vi "sum of N Gaussians with offset model_MODCA.vi"(3 "output control":T1, 4 "data":variant, 5 "X":dbl[](array[numeric]), 6 "a":dbl[](array[numeric])) -> (0 "error out":errorcluster, 1 "f'(X,a)":dbl[][](array[numeric]), 2 "f(X,a)":dbl[](array[numeric]))   [LabVIEW 2020]
doc: "Sum of three Gaussians, plus DC offset."
uses:
  <vilib>/gmath/NumericalOptimization/LM_output select.ctl
  <vilib>/gmath/NI_Gmath.lvlib
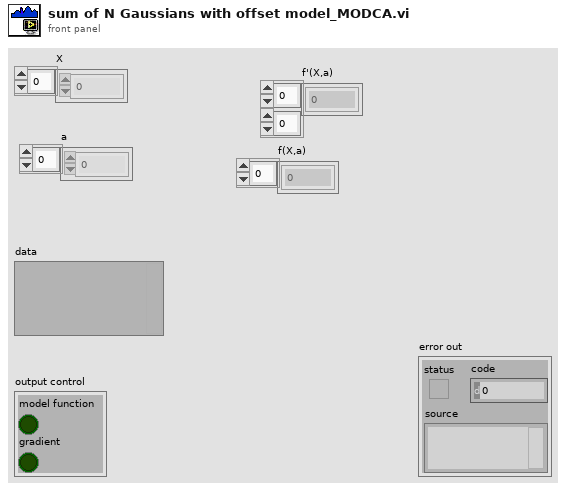
[diagram p1: front panel]
types:
  T1 = typedef "NI_Gmath.lvlib/LM_output select.ctl" = cluster{"model function":bool, "gradient":bool}
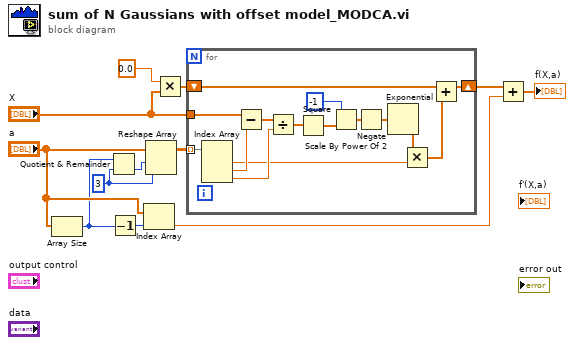
[diagram p0: block diagram]
diagram:
  w4 = 3 ("y")
  n1 = Array Size(array="a") -> (size(s)=w11:i32)
  n2 = Quotient & Remainder(x=w11, y=w4) -> (floor(x/y)=w3:i32)  [unwired: 1 out]
  n3 = Decrement(x=w11) -> (x-1=w6:i32)
  n4 = Index Array(array="a", index=w6) -> (element=w7:dbl)
  n5 = Reshape Array("a", w3, w4) -> (w5:dbl[][])
  n6 = Multiply(x=0.0 ("element"), y="X") -> (x*y=w9:dbl[])
  n7 = for {
    tunnel: w5 -> [w27] mode=indexing
    tunnel: "X" -> [w22]
    shift-right: [w19] -> w8
    shift-left: w9 -> [w21]
    n8 = Index Array(array=w27) -> (element #1=w18:dbl, element #2=w24:dbl, element #3=w23:dbl)  [unwired: 3 in]
    n9 = Subtract(x=w22, y=w24) -> (x-y=w26:dbl[])
    n10 = Divide(x=w26, y=w23) -> (x/y=w25:dbl[])
    n11 = Square(x=w25) -> (x^2=w15:dbl[])
    n12 = Scale By Power Of 2(n=i16 -1, x=w15) -> (x*2^n=w16:dbl[])
    n13 = Negate(x=w16) -> (-x=w13:dbl[])
    n14 = Exponential(1:w13) -> (0:w17:dbl[])
    n15 = Multiply(x=w17, y=w18) -> (x*y=w20:dbl[])
    n16 = Add(x=w21, y=w20) -> (x+y=w19:dbl[])
  }
  n17 = Add(x=w8, y=w7) -> (x+y=→"f(X,a)":dbl[])
